vi "flatsequence.vi"() -> ()   [LabVIEW 2016]
panel:
  out "x-y 2":dbl
  out "Triangle 2":dynamicdata(graph) caption="Triangle"
  out "Sine 2":dynamicdata(graph) caption="Sine"
  out "x-y":dbl
  out "Triangle":dynamicdata(graph)
  out "Sine":dynamicdata(graph)
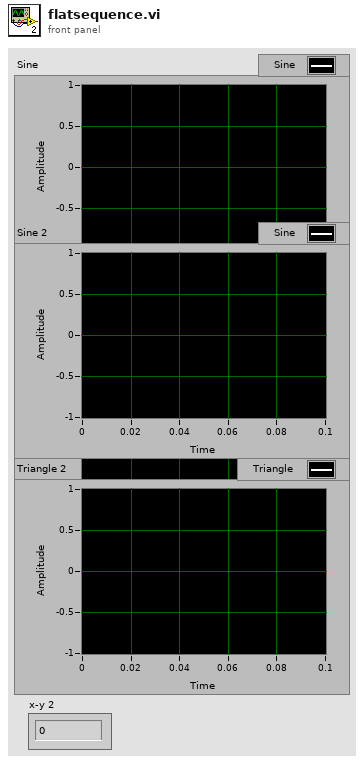
[diagram p1: front panel]
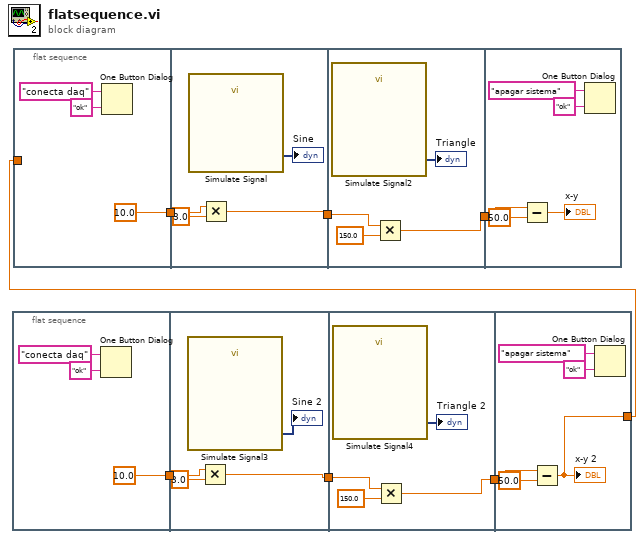
[diagram p0: block diagram]
diagram:
  n1 = flat-sequence {
    tunnel: [10.0] -> w4
    tunnel: w4 -> [w13]
    tunnel: [w11] -> w3
    tunnel: w3 -> [w16]
    tunnel: [w15] -> w2
    tunnel: w2 -> [w21]
    tunnel: [w19] -> w1
    frame #0 {
      n2 = One Button Dialog(message="conecta daq", button name ("OK")="ok") -> ()  [unwired: 1 out]
    }
    frame #1 {
      n3 = call "Simulate Signal3"() -> ("Sine"=→"Sine 2":dynamicdata)  [unwired: 14 in, 1 out]
      n4 = Multiply(x=w13, y=3.0) -> (x*y=w11:dbl)
    }
    frame #2 {
      n5 = call "Simulate Signal4"() -> ("Triangle"=→"Triangle 2":dynamicdata)  [unwired: 14 in, 1 out]
      n6 = Multiply(x=w16, y=150.0) -> (x*y=w15:dbl)
    }
    frame #3 {
      n7 = Subtract(x=w21, y=50.0) -> (x-y=w19:dbl)
      "x-y 2" <- w19
      n8 = One Button Dialog(message="apagar sistema", button name ("OK")="ok") -> ()  [unwired: 1 out]
    }
  }
  n9 = flat-sequence {
    tunnel: [10.0] -> w7
    tunnel: w1 -> [_]
    tunnel: w7 -> [w29]
    tunnel: [w27] -> w6
    tunnel: w6 -> [w32]
    tunnel: [w31] -> w5
    tunnel: w5 -> [w37]
    frame #0 {
      n10 = One Button Dialog(message="conecta daq", button name ("OK")="ok") -> ()  [unwired: 1 out]
    }
    frame #1 {
      n11 = call "Simulate Signal"() -> ("Sine"=→"Sine":dynamicdata)  [unwired: 14 in, 1 out]
      n12 = Multiply(x=w29, y=3.0) -> (x*y=w27:dbl)
    }
    frame #2 {
      n13 = call "Simulate Signal2"() -> ("Triangle"=→"Triangle":dynamicdata)  [unwired: 14 in, 1 out]
      n14 = Multiply(x=w32, y=150.0) -> (x*y=w31:dbl)
    }
    frame #3 {
      n15 = Subtract(x=w37, y=50.0) -> (x-y=→"x-y":dbl)
      n16 = One Button Dialog(message="apagar sistema", button name ("OK")="ok") -> ()  [unwired: 1 out]
    }
  }
